vi "deinterlace.vi"(4 "Scan trap 3 or Fl?":bool=TRUE, 5 "Detector type":string, 6 "Data":i16[](array[numeric]), 7 "Trap sets":u32, 8 "Flip x sign":bool) -> (0 "Channel pattern":i32, 1 "Channel names":string[](array[string]), 2 "Deinterlaced normalized data":dbl[][](array[numeric]), 3 "Deinterlaced data":i16[](array[numeric]))   [LabVIEW 2014]
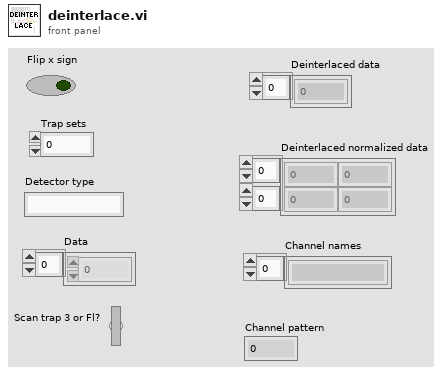
[diagram p1: front panel]
types:
  T1 = cluster{string, string, string, string, string, string, string, string}
  T2 = cluster{string, string, string, string, string, string, string, string, string, string, string, string}
  T3 = cluster{string, string, string, string, string, string, string, string, string, string, string, string, string}
  T4 = cluster{string, string, string, string, string, string, string, string, string, string, string, string, string, string}
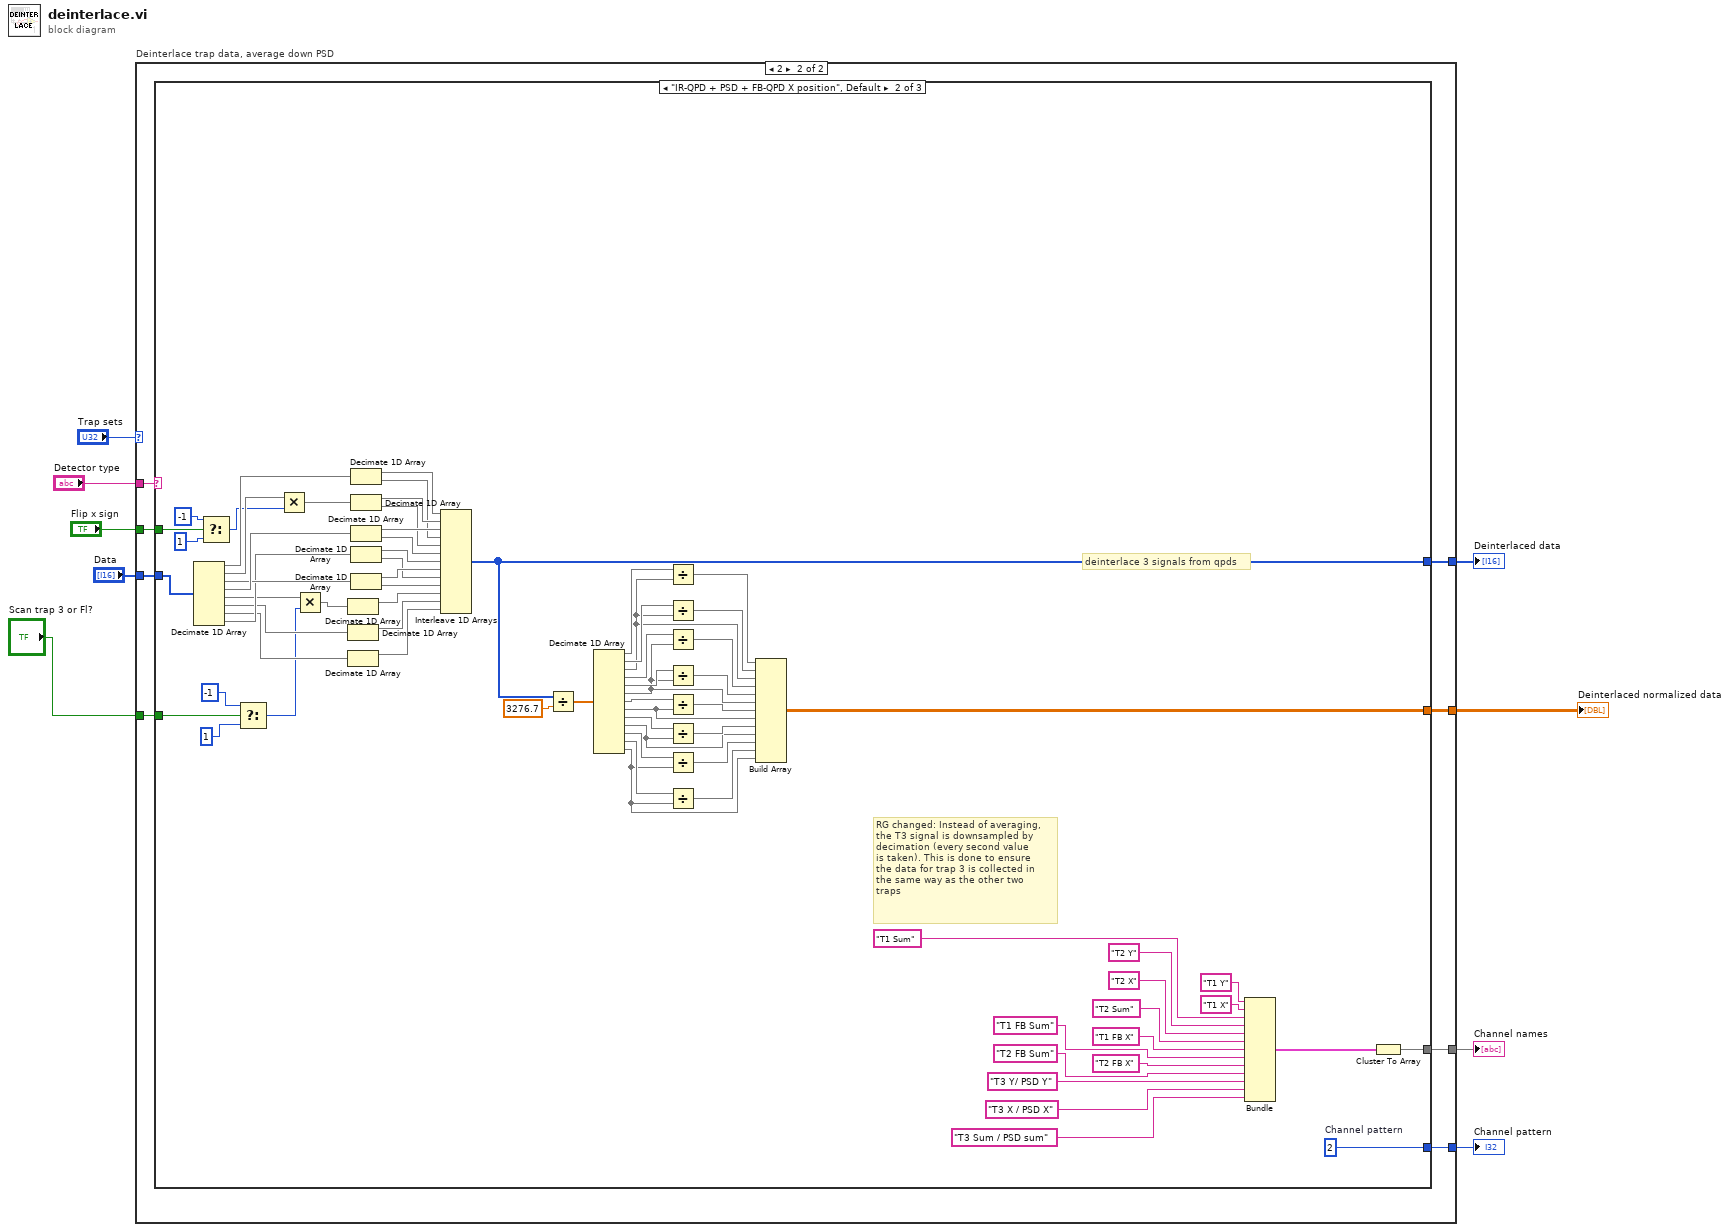
[diagram p0: block diagram]
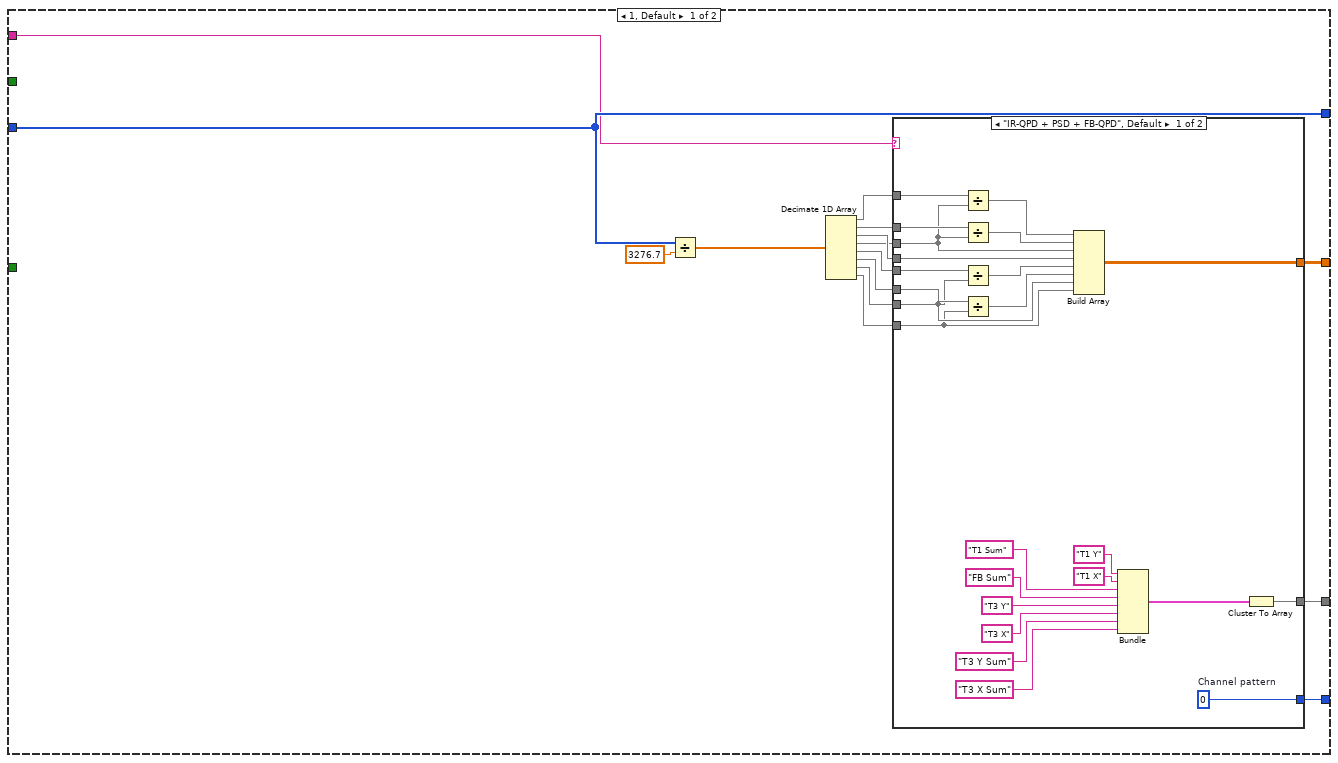
[diagram p2: hidden frame]
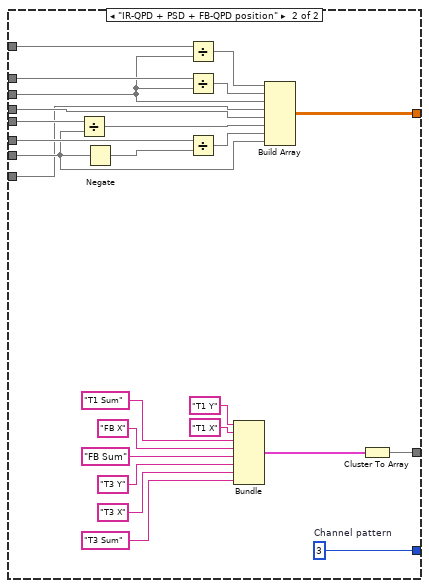
[diagram p3: hidden frame]
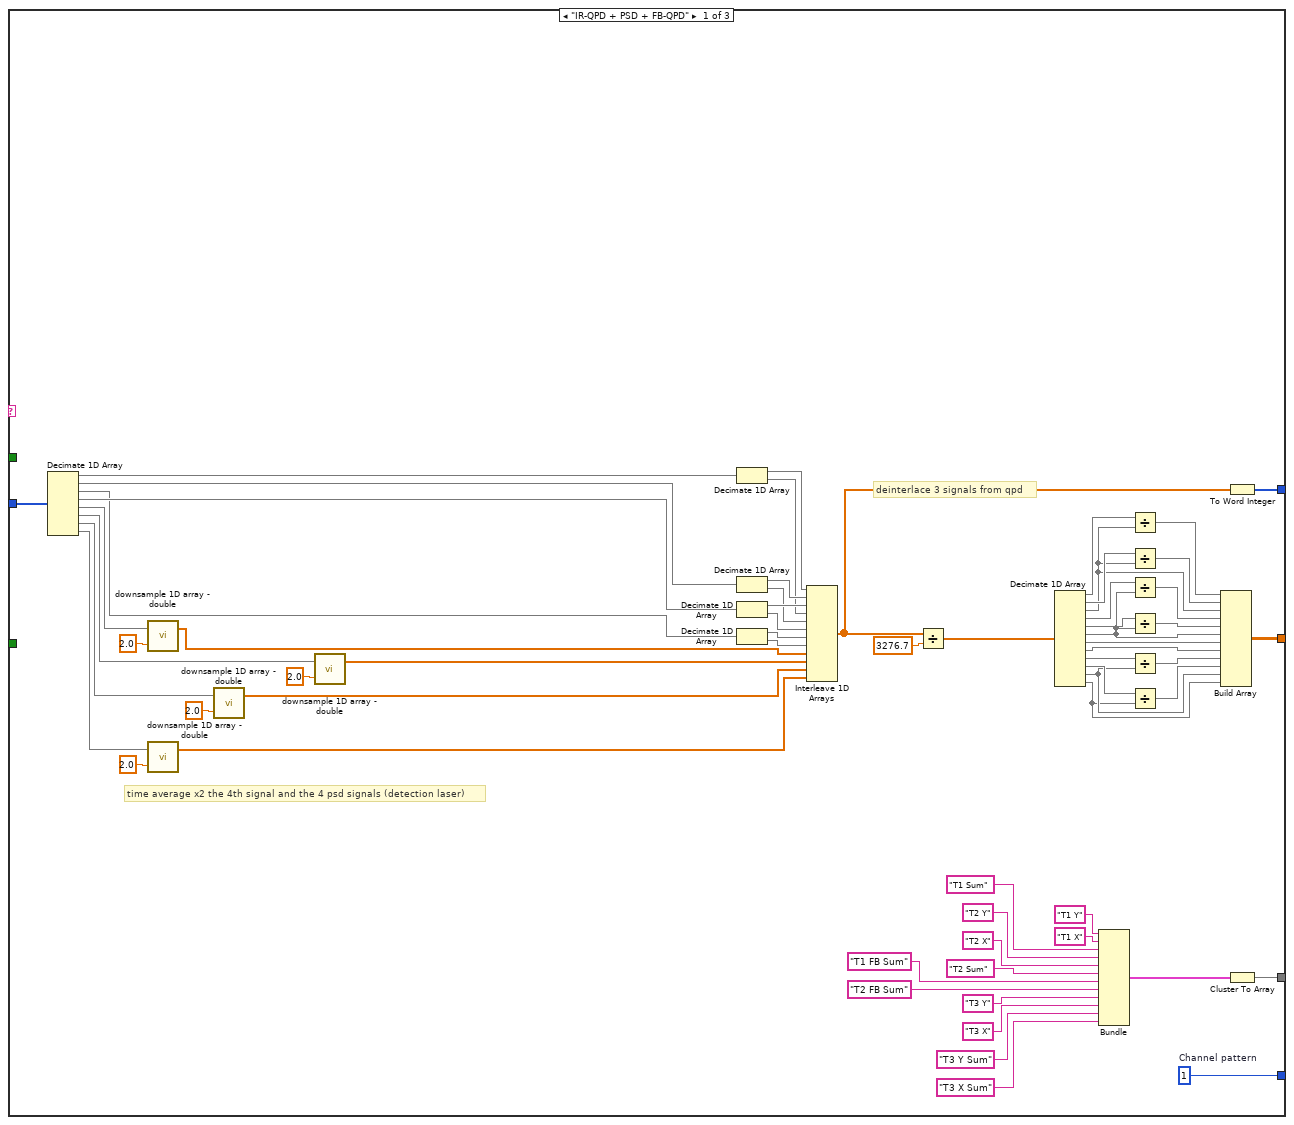
[diagram p4: hidden frame]
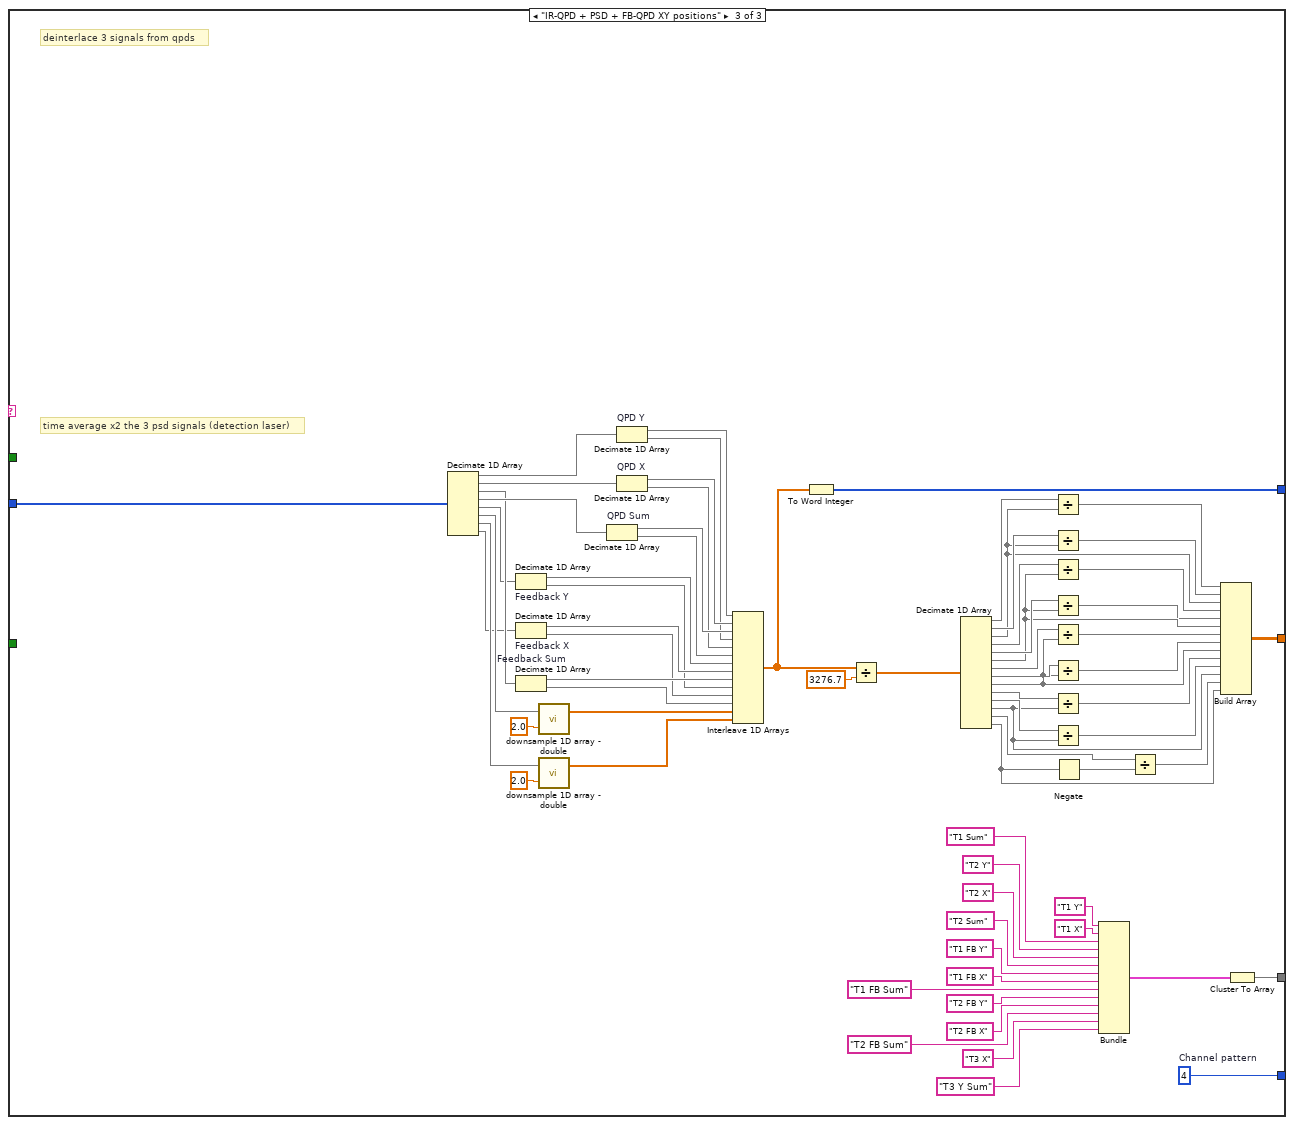
[diagram p5: hidden frame]
diagram:
  n1 = case "Deinterlace trap data, average down PSD" shown="2" "Trap sets" {
    tunnel: "Data" -> [w14 w81]
    tunnel: [w11 w78] -> w4
    tunnel: [w14 w80] -> w5
    tunnel: "Detector type" -> [w13 w76]
    tunnel: [w12 w79] -> w3
    tunnel: [w10 w77] -> w2
    tunnel: "Flip x sign" -> [_ w75]
    tunnel: "Scan trap 3 or Fl?" -> [_ w74]
    frame 1, Default {
      n2 = Divide(x=w14, y=3276.7) -> (x/y=w15:dbl[])
      n3 = Decimate 1D Array(w15) -> (w24:dbl[], w23:dbl[], w22:dbl[], w21:dbl[], w20:dbl[], w19:dbl[], w18:dbl[], w17:dbl[])
      n4 = case shown="\"IR-QPD + PSD + FB-QPD\", Default" w13 {
        tunnel: w24 -> [w48 w73]
        tunnel: w23 -> [w47 w72]
        tunnel: w22 -> [w32 w50]
        tunnel: w21 -> [w33 w60]
        tunnel: w20 -> [w46 w71]
        tunnel: w19 -> [w45 w70]
        tunnel: w18 -> [w29 w51]
        tunnel: w17 -> [w28 w49]
        tunnel: [w27 w57] -> w12
        tunnel: [w26 w56] -> w11
        tunnel: [w25 w55] -> w10
        frame "IR-QPD + PSD + FB-QPD", Default {
          w25 = 0  # Channel pattern
          n5 = Divide(x=w48, y=w33) -> (x/y=w35:dbl[])
          n6 = Divide(x=w47, y=w33) -> (x/y=w34:dbl[])
          n7 = Divide(x=w46, y=w29) -> (x/y=w31:dbl[])
          n8 = Divide(x=w45, y=w28) -> (x/y=w30:dbl[])
          n9 = Build Array(w35, w34, w33, w32, w31, w30, w29, w28) -> (w26:dbl[][])
          n10 = Bundle("T1 Y", "T1 X", "T1 Sum", "FB Sum", "T3 Y", "T3 X", "T3 Y Sum", "T3 X Sum") -> (w44:T1)  [unwired: 1 out]
          n11 = Cluster To Array(cluster=w44) -> (array=w27:string[])
        }
        frame "IR-QPD + PSD + FB-QPD position" {
          w55 = 3  # Channel pattern
          n12 = Divide(x=w71, y=w51) -> (x/y=w59:dbl[])
          n13 = Negate(x=w51) -> (-x=w52:dbl[])
          n14 = Divide(x=w73, y=w60) -> (x/y=w62:dbl[])
          n15 = Divide(x=w72, y=w60) -> (x/y=w61:dbl[])
          n16 = Divide(x=w70, y=w52) -> (x/y=w58:dbl[])
          n17 = Bundle("T1 Y", "T1 X", "T1 Sum", "FB X", "FB Sum", "T3 Y", "T3 X", "T3 Sum") -> (w69:T1)  [unwired: 1 out]
          n18 = Build Array(w62, w61, w60, w49, w50, w59, w58, w51) -> (w56:dbl[][])
          n19 = Cluster To Array(cluster=w69) -> (array=w57:string[])
        }
      }
    }
    frame 2 {
      n20 = case shown="\"IR-QPD + PSD + FB-QPD X position\", Default" w76 {
        tunnel: w81 -> [w143 w216 w287]
        tunnel: [w82 w207 w218] -> w80
        tunnel: [w109 w198 w265] -> w79
        tunnel: [w108 w162 w232] -> w78
        tunnel: [w102 w196 w263] -> w77
        tunnel: w75 -> [_ w157 _]
        tunnel: w74 -> [_ w148 _]
        frame "IR-QPD + PSD + FB-QPD" {
          w102 = 1  # Channel pattern
          # "time average x2 the 4th signal and the 4 psd signals (detection laser)"
          # "deinterlace 3 signals from qpd"
          n21 = Decimate 1D Array(w143) -> (w142:i16[], w141:i16[], w107:i16[], w140:i16[], w130:i16[], w128:i16[], w127:i16[], w125:i16[])
          n22 = call "downsample 1D array - double.vi"("Ave N"=2.0, "Array In"=w130) -> ("Array Out"=w129:dbl[])  [unwired: 1 out]
          n23 = call "downsample 1D array - double.vi"("Ave N"=2.0, "Array In"=w125) -> ("Array Out"=w124:dbl[])  [unwired: 1 out]
          n24 = call "downsample 1D array - double.vi"("Ave N"=2.0, "Array In"=w127) -> ("Array Out"=w126:dbl[])  [unwired: 1 out]
          n25 = call "downsample 1D array - double.vi"("Ave N"=2.0, "Array In"=w128) -> ("Array Out"=w110:dbl[])  [unwired: 1 out]
          n26 = Decimate 1D Array(w142) -> (w139:i16[], w111:i16[])
          n27 = Decimate 1D Array(w141) -> (w138:i16[], w136:i16[])
          n28 = Decimate 1D Array(w140) -> (w137:i16[], w135:i16[])
          n29 = Decimate 1D Array(w107) -> (w106:i16[], w105:i16[])
          n30 = Interleave 1D Arrays(w139, w138, w137, w111, w136, w135, w106, w105, w129, w110, w126, w124) -> (w123:dbl[])
          n31 = Divide(x=w123, y=3276.7) -> (x/y=w122:dbl[])
          n32 = Decimate 1D Array(w122) -> (w121:dbl[], w120:dbl[], w119:dbl[], w118:dbl[], w117:dbl[], w116:dbl[], w104:dbl[], w103:dbl[], w115:dbl[], w114:dbl[], w113:dbl[], w112:dbl[])
          n33 = Bundle("T1 Y", "T1 X", "T1 Sum", "T2 Y", "T2 X", "T2 Sum", "T1 FB Sum", "T2 FB Sum", "T3 Y", "T3 X", "T3 Y Sum", "T3 X Sum") -> (w90:T2)  [unwired: 1 out]
          n34 = Divide(x=w121, y=w119) -> (x/y=w89:dbl[])
          n35 = Divide(x=w120, y=w119) -> (x/y=w88:dbl[])
          n36 = Divide(x=w118, y=w116) -> (x/y=w87:dbl[])
          n37 = Divide(x=w117, y=w116) -> (x/y=w86:dbl[])
          n38 = Divide(x=w115, y=w113) -> (x/y=w85:dbl[])
          n39 = Divide(x=w114, y=w112) -> (x/y=w84:dbl[])
          n40 = Build Array(w89, w88, w119, w87, w86, w116, w104, w103, w85, w84, w113, w112) -> (w108:dbl[][])
          n41 = To Word Integer(number=w123) -> (16bit integer=w82:i16[])
          n42 = Cluster To Array(cluster=w90) -> (array=w109:string[])
        }
        frame "IR-QPD + PSD + FB-QPD X position", Default {
          w196 = 2  # Channel pattern
          # "RG changed: Instead of averaging,\nthe T3 signal is downsampled by \ndecimation (every second value\nis taken). This is done to ensure\nthe data for trap 3 is collected in \nthe same way as the other two \ntraps"
          # "deinterlace 3 signals from qpds"
          n43 = Decimate 1D Array(w216) -> (w215:i16[], w214:i16[], w197:i16[], w213:i16[], w147:i16[], w151:i16[], w156:i16[], w184:i16[])
          n44 = Select(t=i16 -1, s=w157, f=i16 1) -> (s? t:f=w160:i16)
          n45 = Select(t=i16 -1, s=w148, f=i16 1) -> (s? t:f=w146:i16)
          n46 = Multiply(x=w214, y=w160) -> (x*y=w161:i16[])
          n47 = Multiply(x=w147, y=w146) -> (x*y=w145:i16[])
          n48 = Decimate 1D Array(w145) -> (w153:i16[])  [unwired: 1 out]
          n49 = Decimate 1D Array(w151) -> (w154:i16[])  [unwired: 1 out]
          n50 = Decimate 1D Array(w156) -> (w155:i16[])  [unwired: 1 out]
          n51 = Decimate 1D Array(w215) -> (w212:i16[], w199:i16[])
          n52 = Decimate 1D Array(w161) -> (w211:i16[], w209:i16[])
          n53 = Decimate 1D Array(w213) -> (w210:i16[], w208:i16[])
          n54 = Decimate 1D Array(w184) -> (w183:i16[], w181:i16[])
          n55 = Decimate 1D Array(w197) -> (w182:i16[], w180:i16[])
          n56 = Interleave 1D Arrays(w212, w211, w210, w199, w209, w208, w183, w182, w181, w180, w153, w154, w155) -> (w207:i16[])
          n57 = Divide(x=w207, y=3276.7) -> (x/y=w206:dbl[])
          n58 = Decimate 1D Array(w206) -> (w205:dbl[], w204:dbl[], w203:dbl[], w202:dbl[], w201:dbl[], w200:dbl[], w172:dbl[], w170:dbl[], w169:dbl[], w167:dbl[], w166:dbl[], w165:dbl[], w152:dbl[])
          n59 = Divide(x=w205, y=w203) -> (x/y=w188:dbl[])
          n60 = Divide(x=w204, y=w203) -> (x/y=w187:dbl[])
          n61 = Divide(x=w202, y=w200) -> (x/y=w186:dbl[])
          n62 = Divide(x=w201, y=w200) -> (x/y=w185:dbl[])
          n63 = Divide(x=w172, y=w170) -> (x/y=w171:dbl[])
          n64 = Divide(x=w169, y=w167) -> (x/y=w168:dbl[])
          n65 = Divide(x=w166, y=w152) -> (x/y=w164:dbl[])
          n66 = Divide(x=w165, y=w152) -> (x/y=w163:dbl[])
          n67 = Build Array(w188, w187, w203, w186, w185, w200, w171, w170, w168, w167, w164, w163, w152) -> (w162:dbl[][])
          n68 = Bundle("T1 Y", "T1 X", "T1 Sum", "T2 Y", "T2 X", "T2 Sum", "T1 FB X", "T1 FB Sum", "T2 FB X", "T2 FB Sum", "T3 Y/ PSD Y", "T3 X / PSD X", "T3 Sum / PSD sum") -> (w189:T3)  [unwired: 1 out]
          n69 = Cluster To Array(cluster=w189) -> (array=w198:string[])
        }
        frame "IR-QPD + PSD + FB-QPD XY positions" {
          w263 = 4  # Channel pattern
          # "time average x2 the 3 psd signals (detection laser)"
          # "deinterlace 3 signals from qpds"
          n70 = Decimate 1D Array(w287) -> (w286:i16[], w285:i16[], w264:i16[], w284:i16[], w230:i16[], w276:i16[], w275:i16[], w252:i16[])
          n71 = Decimate 1D Array "Feedback Y"(w230) -> (w229:i16[], w228:i16[])
          n72 = Decimate 1D Array "Feedback X"(w252) -> (w249:i16[], w247:i16[])
          n73 = Decimate 1D Array "Feedback Sum"(w264) -> (w248:i16[], w246:i16[])
          n74 = call "downsample 1D array - double.vi"("Ave N"=2.0, "Array In"=w276) -> ("Array Out"=w251:dbl[])  [unwired: 1 out]
          n75 = call "downsample 1D array - double.vi"("Ave N"=2.0, "Array In"=w275) -> ("Array Out"=w250:dbl[])  [unwired: 1 out]
          n76 = Decimate 1D Array "QPD Sum"(w284) -> (w281:i16[], w279:i16[])
          n77 = Decimate 1D Array "QPD Y"(w286) -> (w283:i16[], w266:i16[])
          n78 = Decimate 1D Array "QPD X"(w285) -> (w282:i16[], w280:i16[])
          n79 = Interleave 1D Arrays(w283, w282, w281, w266, w280, w279, w229, w249, w248, w228, w247, w246, w251, w250) -> (w274:dbl[])
          n80 = To Word Integer(number=w274) -> (16bit integer=w218:i16[])
          n81 = Divide(x=w274, y=3276.7) -> (x/y=w273:dbl[])
          n82 = Decimate 1D Array(w273) -> (w272:dbl[], w271:dbl[], w270:dbl[], w269:dbl[], w268:dbl[], w267:dbl[], w225:dbl[], w239:dbl[], w223:dbl[], w224:dbl[], w237:dbl[], w221:dbl[], w235:dbl[], w233:dbl[])
          n83 = Divide(x=w272, y=w270) -> (x/y=w256:dbl[])
          n84 = Divide(x=w271, y=w270) -> (x/y=w255:dbl[])
          n85 = Divide(x=w269, y=w267) -> (x/y=w254:dbl[])
          n86 = Divide(x=w268, y=w267) -> (x/y=w253:dbl[])
          n87 = Divide(x=w225, y=w223) -> (x/y=w222:dbl[])
          n88 = Divide(x=w239, y=w223) -> (x/y=w238:dbl[])
          n89 = Divide(x=w224, y=w221) -> (x/y=w220:dbl[])
          n90 = Divide(x=w237, y=w221) -> (x/y=w236:dbl[])
          n91 = Negate(x=w233) -> (-x=w231:dbl[])
          n92 = Bundle("T1 Y", "T1 X", "T1 Sum", "T2 Y", "T2 X", "T2 Sum", "T1 FB Y", "T1 FB X", "T1 FB Sum", "T2 FB Y", "T2 FB X", "T2 FB Sum", "T3 X", "T3 Y Sum") -> (w219:T4)  [unwired: 1 out]
          n93 = Divide(x=w235, y=w231) -> (x/y=w234:dbl[])
          n94 = Build Array(w256, w255, w270, w254, w253, w267, w222, w238, w223, w220, w236, w221, w234, w233) -> (w232:dbl[][])
          n95 = Cluster To Array(cluster=w219) -> (array=w265:string[])
        }
      }
    }
  }
  "Deinterlaced data" <- w5
  "Deinterlaced normalized data" <- w4
  "Channel names" <- w3
  "Channel pattern" <- w2
